vi "example.vi"(8 "Message":string, 9 "Title":string, 10 "Group":string, 11 "urls":string[](array[string])) -> ()   [LabVIEW 2016]
uses:
  Bark/Bark.lvclass
  Bark/Bark.lvclass/Bark.ctl
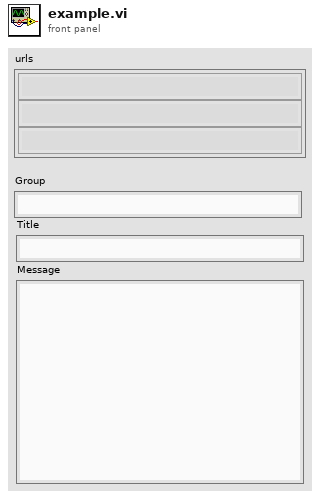
[diagram p1: front panel]
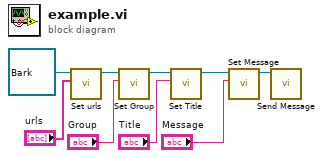
[diagram p0: block diagram]
diagram:
  n1 = call "Set urls.vi"("urls"="urls", "Bark in"=refnum<class "Bark.lvclass"> refnum ("Bark.lvlib:Bark.lvclass")) -> ("Bark out"=w8:refnum<class "Bark.lvclass">)  [unwired: 9 in]
  n2 = call "Set Group.vi"("Group"="Group", "Bark in"=w8) -> ("Bark out"=w7:refnum<class "Bark.lvclass">)  [unwired: 9 in]
  n3 = call "Set Title.vi"("Title"="Title", "Bark in"=w7) -> ("Bark out"=w6:refnum<class "Bark.lvclass">)  [unwired: 9 in]
  n4 = call "Set Message.vi"("Message"="Message", "Bark in"=w6) -> ("Bark out"=w5:refnum<class "Bark.lvclass">)  [unwired: 9 in]
  n5 = call "Send Message.vi"("Bark 输入"=w5) -> ()  [unwired: 9 in, 2 out]
